vi "GVTrapsMachs_ECD.vi"() -> ()   [LabVIEW 2017]
panel:
  in  "Traps/Machs":dbl[](array[numeric])
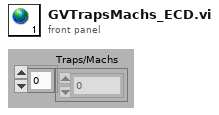
[diagram p1: front panel]
diagram:
